vi "UHR-Fleezers Control (host) - Lorentz v2.vi"() -> ()   [LabVIEW 2014] (continued)
          n51 = call "Close.vi"("error in (no error)"=w127, "TTL in"=w124) -> ("error out"=w122:errorcluster)  [unwired: 8 in, 1 out]
        }
        frame Error {
          n52 = call <vilib>:"Simple Error Handler.vi"("error in (no error)"=w205) -> ("error out"=w204:errorcluster)  [unwired: 4 in, 4 out]
        }
      }
      n53 = property on="DAQmx Device Name" class="DAQmxName"("Visible"=FALSE) -> ()  [unwired: 2 in, 2 out]
      n54 = call <vilib>:"Clear Errors.vi"("error in (no error)"=w89) -> ("error out"=w87:errorcluster)  [unwired: 5 in, 1 out]
      n55 = property on="DAQmx Device Name" class="DAQmxName"(error in=w87, "Visible"=TRUE) -> ()  [unwired: 1 in, 2 out]
    }
    frame Disabled {
    }
  }
  n56 = xnode "Open FPGA VI Reference"("resource name"=T24 "RIO0") -> ("FPGA VI Reference Out"=w26:T31, "error out"=w25:errorcluster)  [unwired: 1 in]
  n57 = xnode "Invoke Method"("FPGA VI Reference In"=w26, "error in"=w25) -> ("FPGA VI Reference Out"=w6:T31, "error out"=→"FPGA error out":errorcluster)
  n58 = Subtract(x=w4, y="Maximum Delta\n(MHz)") -> (x-y=w2:dbl)
  n59 = Bundle By Name(cluster=T20 {"Minimum"=60.0, "Maximum"=90.0, "Increment"=1.0} ("Min Max Inc"), "Minimum"=w2, "Maximum"=w4) -> (w1:T20)
  n60 = flat-sequence "Safety limits on RF frequencies and amplitudes (for AOM protection)" {
    tunnel: [w208] -> w17
    tunnel: [w206] -> w19
    tunnel: [w209] -> w20
    tunnel: [w210] -> w18
    tunnel: w1 -> [w208]
    tunnel: T20 {"Minimum"=0.0, "Maximum"=50.0, "Increment"=1.0} ("Data Entry Limits") -> [w206]
    tunnel: w6 -> [w207]
    tunnel: [w207] -> w21
    frame #0 {
      w210 = T20 {"Minimum"=0.0, "Maximum"=40.0, "Increment"=0.1} ("Min Max Inc")
      w209 = T20 {"Minimum"=0.0, "Maximum"=45.0, "Increment"=1.0} ("Data Entry Limits")
      n61 = property on="BD 2 Frequency 1 (MHz)" class="DigNum (strict)"("Data Range"=w210) -> ()  [unwired: 2 in, 2 out]
      n62 = property on="BD 2 Frequency 3 (MHz)" class="DigNum (strict)"("Data Range"=w210) -> ()  [unwired: 2 in, 2 out]
      n63 = property on="BD 2 Frequency 2 (MHz)" class="DigNum (strict)"("Data Range"=w210) -> ()  [unwired: 2 in, 2 out]
      n64 = property on="BD 1 Frequency 1 (MHz)" class="DigNum (strict)"("Data Range"=w208) -> ()  [unwired: 2 in, 2 out]
      n65 = property on="BD 1 Frequency 2 (MHz)" class="DigNum (strict)"("Data Range"=w208) -> ()  [unwired: 2 in, 2 out]
      n66 = property on="BD 1 Frequency 3 (MHz)" class="DigNum (strict)"("Data Range"=w208) -> ()  [unwired: 2 in, 2 out]
      n67 = property on="BD 2 Amplitude 1 (%)" class="DigNum (strict)"("Data Range"=w209) -> ()  [unwired: 2 in, 2 out]
      n68 = property on="BD 2 Amplitude 2 (%)" class="DigNum (strict)"("Data Range"=w209) -> ()  [unwired: 2 in, 2 out]
      n69 = property on="BD 2 Amplitude 3 (%)" class="DigNum (strict)"("Data Range"=w209) -> ()  [unwired: 2 in, 2 out]
      n70 = property on="BD 1 Amplitude 3 (%)" class="DigNum (strict)"("Data Range"=w206) -> ()  [unwired: 2 in, 2 out]
      n71 = property on="BD 1 Amplitude 2 (%)" class="DigNum (strict)"("Data Range"=w206) -> ()  [unwired: 2 in, 2 out]
      n72 = property on="BD 1 Amplitude 1 (%)" class="DigNum (strict)"("Data Range"=w206) -> ()  [unwired: 2 in, 2 out]
      "X RF Frequency Limits (MHz)" <- w208
      "X RF Amplitude Limits (%)" <- w206
      "Y RF Amplitude Limits (%)" <- w209
      "Y RF Frequency Limits (MHz)" <- w210
    }
  }
  n73 = stacked-sequence "Host initialization sequence - order matters!" {
    tunnel: w21 -> [_ w230 w322 _ w379 w388 w455 w479 _ w513]
    tunnel: [_ _ _ _ _ _ _ _ _ w513] -> w10
    tunnel: [_ _ _ _ _ _ _ _ _ w512] -> w23
    tunnel: w20 -> [_ _ _ _ _ _ w453 _ _ _]
    tunnel: w19 -> [_ _ _ _ _ _ w452 _ _ _]
    tunnel: w18 -> [_ _ _ _ _ _ w451 _ _ _]
    tunnel: w17 -> [_ _ _ _ _ _ w432 _ _ _]
    tunnel: [_ _ _ _ _ _ _ _ w507 _] -> _
    frame #0 {
    }
    frame #1 {
      w262 = 10.0 ("y")
      w263 = 32767.0 ("y")
      w247 = 6.0  # clock mult.
      w246 = 49152000.0  # TCXO frequ.
      # "Initialize some FPGA settings"
      n74 = local read "Not-Interlacing Set"() -> (w302:enum32{"Set 1", "Set 2", "Set 3"})
      n75 = local write "Trap Pos FIFO Timeout"(u16 0 ("Trap Pos FIFO Timeout")) -> ()
      n76 = local read "Interlace"() -> (w300:bool)
      n77 = local read "Desired Scan Incr (V)"() -> (w274:dbl)
      n78 = local read "BD 1 Delay (ticks)"() -> (w309:u8)
      n79 = local read "Number Interlace Sets"() -> (w301:u8)
      n80 = local read "BD 2 Delay (Ticks)"() -> (w310:u8)
      n81 = property on="AI Count (ticks)" class="DigNum (strict)"("Val(Sgnl)"="AI Count (ticks)") -> ()  [unwired: 2 in, 2 out]
      n82 = local read "AO1"() -> (w268:dbl)
      n83 = local read "AO2"() -> (w269:dbl)
      n84 = local read "Next trap write delay (ticks)"() -> (w311:u8)
      n85 = local read "Number of scans (MCL)"() -> (w278:u64)
      n86 = local read "Cycles/step (MCL)"() -> (w277:u64)
      n87 = local read "Scan steps (MCL)"() -> (w276:u64)
      n88 = local read "Continuous MCL Scanning"() -> (w279:bool)
      n89 = Multiply(x=w268, y=w263) -> (x*y=w266:dbl)
      n90 = Multiply(x=w269, y=w263) -> (x*y=w264:dbl)
      n91 = Build Array("DIO count 1 (ticks)", "DIO count 2 (ticks)", "DIO count 3 (ticks)") -> (w295:u16[])
      n92 = local read "Fast Scan Dir"() -> (w280:bool)
      n93 = local read "2D or 1D Scan"() -> (w292:bool)
      n94 = local read "N Acq Sets (Traps + Fl.)"() -> (w288:i16)
      n95 = local read "Scan Increment (MHz)"() -> (w251:dbl)
      n96 = Divide(x=w266, y=w262) -> (x/y=w267:dbl)
      n97 = Divide(x=w264, y=w262) -> (x/y=w265:dbl)
      n98 = To Unsigned Byte Integer(number=w302) -> (unsigned 8bit integer=w297:u8)
      n99 = Split 1D Array(array=w295, index=w301) -> (first subarray=w293:u16[])  [unwired: 1 out]
      n100 = Multiply(x=w274, y=32767.0) -> (x*y=w272:dbl)
      n101 = To Word Integer(number=w267) -> (16bit integer=w213:i16)
      n102 = To Word Integer(number=w265) -> (16bit integer=w212:i16)
      n103 = Index Array(array=w295, index=w297) -> (element=w296:u16)
      n104 = Add Array Elements(numeric array=w293) -> (sum=w294:u16)
      n105 = Multiply(x=w246, y=w247) -> (x*y=w248:dbl)
      n106 = Divide(x=w272, y=10.0) -> (x/y=w273:dbl)
      n107 = Select(t=w294, s=w300, f=w296) -> (s? t:f=w303:u16)
      n108 = Not(x=w280) -> (.not. x?=w281:bool)
      n109 = To Word Integer(number=w273) -> (16bit integer=w275:i16)
      n110 = property on="2D or 1D Scan" class="Bool (strict)"("Val(Sgnl)"=w292) -> ()  [unwired: 2 in, 2 out]
      n111 = Divide(x=40000000.0, y="AI Count (ticks)") -> (x/y=w284:dbl)
      n112 = local write "Update Count (MCL)"(w303) -> ()
      n113 = local write "Total Counts (ticks)"(w303) -> ()
      n114 = Divide(x=w284, y="FPGA Ave.") -> (x/y=w283:dbl)
      n115 = local write "AI rate (Hz)"(w284) -> ()
      n116 = Multiply(x=w251, y=1000.0) -> (x*y=w244:dbl)
      n117 = local write "Ave. Rate (Hz)"(w283) -> ()
      n118 = Reciprocal(x=w283) -> (1/x=w282:dbl)
      n119 = Scale By Power Of 2(n=48, x=w244) -> (x*2^n=w243:dbl)
      n120 = local write "Ave. Period (s)"(w282) -> ()
      n121 = Divide(x=w243, y=w248) -> (x/y=w249:dbl)
      n122 = To Quad Integer(1:w249) -> (0:w252:i64)
      n123 = local read "Setpoints (V)"() -> (w237:cluster{"Set 1":dbl, "Set 2":dbl})
      n124 = local read "# Samples/channel"() -> (w259:u32)
      n125 = local read "Feedback On/Off"() -> (w234:cluster{"Set 1":bool, "Set 2":bool})
      n126 = local read "T3 Y (V)"() -> (w217:dbl)
      n127 = local read "T3 X (V)"() -> (w216:dbl)
      n128 = local read "Trap intensity output range"() -> (w227:cluster{"Normal High":i16, "Normal Low":i16})
      n129 = local read "All FB On/Off"() -> (w233:bool)
      n130 = local read "Number of F/B Scans (AOD)"() -> (w258:u16)
      n131 = local read "Trap Intensity PID Gains"() -> (w226:T11)
      n132 = local read "Cycles/step (AOD)"() -> (w254:u64)
      n133 = local read "Scan steps (AOD)"() -> (w253:u64)
      n134 = Multiply(x=w253, y=w254) -> (x*y=w255:u64)
      n135 = Multiply(x=w255, y=u64 2) -> (x*y=w257:u64)
      n136 = Multiply(x=w257, y=w258) -> (x*y=w260:u64)
      n137 = Multiply(x=3276.7, y=w237) -> (x*y=w238:cluster{"Set 1":dbl, "Set 2":dbl})
      n138 = local read "Scan BD"() -> (w242:bool)
      n139 = Multiply(x=w217, y=32767.0) -> (x*y=w223:dbl)
      n140 = And(x=w234, y=w233) -> (x .and. y?=w235:cluster{"Set 1":bool, "Set 2":bool})
      n141 = To Word Integer(number=w238) -> (16bit integer=w239:cluster{"Set 1":i16, "Set 2":i16})
      n142 = Multiply(x=w216, y=32767.0) -> (x*y=w220:dbl)
      n143 = local read "Sets to FIFO (Traps)"() -> (w305:T19)
      n144 = Divide(x=w260, y=w259) -> (x/y=w261:dbl)
      n145 = Unbundle By Name(w235) -> ("Set 1"=w231:bool, "Set 2"=w232:bool)
      n146 = Unbundle By Name(w239) -> ("Set 1"=w240:i16, "Set 2"=w241:i16)
      n147 = Divide(x=w223, y=10.0) -> (x/y=w224:dbl)
      n148 = Divide(x=w220, y=10.0) -> (x/y=w219:dbl)
      n149 = To Word Integer(number=w224) -> (16bit integer=w215:i16)
      n150 = To Word Integer(number=w219) -> (16bit integer=w214:i16)
      n151 = local read "FPGA error out"() -> (w229:errorcluster)
      n152 = local write "Data points/scan (f/b)"(w257) -> ()
      n153 = local write "Data points/scans"(w260) -> ()
      n154 = local write "N sets should be saved"(w261) -> ()
      n155 = Unbundle By Name(w305) -> ("Set 1"=w306:bool, "Set 2"=w307:bool, "Set 3"=w308:bool)
      n156 = xnode "Read/Write Control"("FPGA VI Reference In"=w230, "error in"=w229, "ai count"="AI Count (ticks)", "Interlace ON/OFF"=w300, "Number Interlace Cycles"=w301, "Set 1"=w306, "Set 2"=w307, "Set 3"=w308, "FB On/Off Set 1"=w231, "FB On/Off Set 2"=w232, "Interlace Off Parameters"=w302, "FB Setpoint Set 1"=w240, "FB Setpoint Set 2"=w241, "AO4"=w215, "AO5"=w214, "FB Gains"=w226, "FB output range"=w227, "Cycles per step"=w254, "Scan BD"=w242, "Number of scans"=w258, "Scan steps"=w253, "Scan freq.  increment"=w252, "AO1"=w213, "AO2"=w212, "Scan freq.  increment (MCL)"=w275, "Scan steps (MCL)"=w276, "Cycles per step (MCL)"=w277, "Number of scans (MCL)"=w278, "MCL count"=w303, "Cont. Scan (MCL)"=w279, "MCL Scan Axis"=w281, "1D or 2D Scan?"=w292, "N of AI1 Int Acq Sets"=w288, "Amp switch delay"="Amp switch delay", "Swap F1 and F2"="Swap F1 and F2", "APD to FIFO"=FALSE, "DIO count 1 (ticks)"="DIO count 1 (ticks)", "DIO count 2 (ticks)"="DIO count 2 (ticks)", "DIO count 3 (ticks)"="DIO count 3 (ticks)", "BD 1 Delay (ticks)"=w309, "BD 2 Delay (Ticks)"=w310, "Next trap write delay (ticks)"=w311) -> ("error out"=w228:errorcluster)  [unwired: 1 out]
      n157 = local write "FPGA error out"(w228) -> ()
    }
    frame #2 {
      # "Initialize some more FPGA settings"
      n158 = local read "Trap Pos FB Monitor\nT1 or T2"() -> (w333:bool)
      n159 = local read "Trap Pos FB Negate Action"() -> (w334:bool)
      n160 = local read "Trap Pos. FB Offset Factor"() -> (w335:i64)
      n161 = local read "Trap Pos. FB Mult Factor"() -> (w336:i64)
      n162 = local read "Trap Pos. AI1 X Pre-scale"() -> (w338:u16)
      n163 = local read "Trap Pos FB Int Count"() -> (w340:u16)
      n164 = local read "Green Laser ON"() -> (w312:bool)
      n165 = local read "Neg. TTrig FPGA"() -> (w341:bool)
      n166 = local read "Trap Pos. FB Range"() -> (w317:T15)
      n167 = local read "Trap Pos. FB Gains"() -> (w318:T14)
      n168 = local read "Dynamic Force FB (ronen)"() -> (w319:bool)
      n169 = Multiply(x="Green Intensity % (FB OFF)", y=655.35) -> (x*y=w327:dbl)
      n170 = Multiply(x="Red FB Setpoint (mV)", y=3.2767) -> (x*y=w349:dbl)
      n171 = Multiply(x="Red Intensity % (FB OFF)", y=655.35) -> (x*y=w353:dbl)
      n172 = Unbundle By Name("Red FB Gains") -> ("proportional gain (Kc)"=w358:i16, "integral gain (Kc*Ts/Ti)"=w359:i16, "derivative gain (Kc*Td/Ts)"=w360:i16)
      n173 = Multiply(x="Green FB Setpoint (mV)", y=3.2767) -> (x*y=w330:dbl)
      n174 = To Unsigned Word Integer(number=w327) -> (unsigned 16bit integer=w329:u16)
      n175 = To Unsigned Word Integer(number=w353) -> (unsigned 16bit integer=w356:u16)
      n176 = To Word Integer(number=w349) -> (16bit integer=w352:i16)
      n177 = local read "Differential FB?"() -> (w343:bool)
      n178 = To Word Integer(number=w330) -> (16bit integer=w332:i16)
      n179 = local read "Laser interlacing mode"() -> (w315:enum32{"Laser ON", "Laser OFF", "Interlace"})
      n180 = local read "Invert laser interlacing"() -> (w316:bool)
      n181 = Unbundle By Name("Green FB Gains") -> ("proportional gain (Kc)"=w346:i16, "integral gain (Kc*Ts/Ti)"=w347:i16, "derivative gain (Kc*Td/Ts)"=w348:i16)
      n182 = Select(t=w315, s=w312, f=enum32{"Laser ON", "Laser OFF", "Interlace"}."Laser OFF" ("Green laser mode")) -> (s? t:f=w314:enum32{"Laser ON", "Laser OFF", "Interlace"})
      n183 = local read "FPGA error out"() -> (w320:errorcluster)
      n184 = xnode "Read/Write Control"("FPGA VI Reference In"=w322, "error in"=w320, "Invert GI"=w316, "Invert GI 2"=w316, "Invert RI"=w316, "Invert RI 2"=w316, "Operating Mode"=w314, "Operating Mode 2"=w314, "Red Laser Operating Mode"=w314, "RI Operating Mode 2"=w314, "P3"=w346, "I3"=w347, "D3"=w348, "Green FB Setpoint"=w332, "Green FB On/Off"="Green FB On/Off", "Current Out"=w329, "Green int current ON count adj"="Green int current ON count adj", "Trap Pos FB Monitor T1 or T2"=w333, "Trap Pos FB Negate Action"=w334, "Trap Pos. FB Offset Factor"=w335, "Trap Pos. FB Mult Factor"=w336, "Force feedback"=FALSE, "AI1 X Scale"=w338, "Trap Pos to FIFO"=TRUE, "Trap Pos FB Int Count"=w340, "TTrig Negate Pos"=w341, "FB Trig Integrate"="FB Trig Integrate", "Diff FB Measurement?"=w343, "Negate Diff?"="Negate Diff?", "Trap pos. FB Range"=w317, "Trap Pos. FB Gains"=w318, "Red FB Setpoint"=w352, "RI Current Out"=w356, "P4"=w358, "I4"=w359, "D4"=w360, "Red FB On/Off"="Red FB On/Off", "Dynamic Force FB (Ronen)"=w319) -> ("error out"=w321:errorcluster)  [unwired: 1 out]
      n185 = local write "FPGA error out"(w321) -> ()
    }
    frame #3 {
      # "Initialize more settings. Should stop using event loops to initialize."
      # "What are these?"
      n186 = local write "Offset (nm)"(0.0 ("Offset (nm)")) -> ()
      n187 = local write "Bead Mean (nm)"(0.0 ("Bead Mean (nm)")) -> ()
      n188 = stacked-sequence {
        frame #0 {
          w364 = T33."empty" ("mode")
          # "Clear external fluorescence triggering FIFO"
          # "APD loop counts"
          # "Fluorescence loop counts (rates)"
          n189 = local read "APD Integration Time (s)"() -> (w366:dbl)
          n190 = local read "Interlace ON count"() -> (w367:u16)
          n191 = call "Smart Buffer (DBL) 1.vi"("mode"=w364) -> ()  [unwired: 5 in, 6 out]
          n192 = call "Smart Buffer (DBL) 2.vi"("mode"=w364) -> ()  [unwired: 5 in, 6 out]
          n193 = property on="APD Integration Time (s)" class="DigNum (strict)"("Val(Sgnl)"=w366) -> ()  [unwired: 2 in, 2 out]
          n194 = property on="Interlace ON count" class="DigNum (strict)"("Val(Sgnl)"=w367) -> ()  [unwired: 2 in, 2 out]
          "Number of APDs" <- 3.0 ("Number of APDs")
        }
        frame #1 {
          # "Number of APDs affects\nAPD DMA transfer"
          # "General settings for all lasers:"
          # "And includes all laser\nON/OFF settings"
          # "Fluorescent lasers settings:"
          # "Blue laser settings:"
          n195 = local read "Laser interlacing mode"() -> (w369:enum32{"Laser ON", "Laser OFF", "Interlace"})
          n196 = local read "Invert laser interlacing"() -> (w368:bool)
          n197 = local read "Blue FB On/Off"() -> (w370:bool)
          n198 = property on="Blue FB On/Off" class="Bool (strict)"("Val(Sgnl)"=w370) -> ()  [unwired: 2 in, 2 out]
          n199 = property on="Invert laser interlacing" class="Bool (strict)"("Val(Sgnl)"=w368) -> ()  [unwired: 2 in, 2 out]
          n200 = property on="Laser interlacing mode" class="RadioBtnsControl (strict)"("Val(Sgnl)"=w369) -> ()  [unwired: 2 in, 2 out]
        }
        frame #2 {
          w371 = path "C:/Home/Bustamante Lab/Comstock-LabView-Link.udl" ("connection information")
          # "Database link changed by Ronen - not clear if it matter for the program."
          # "Initialize the database connection"
          n201 = disable-structure shown="Disabled" {
            disable-tunnel: [w374 _] -> w372
            disable-tunnel: w371 -> [w373 _]
            frame Disabled {
              n202 = call-poly <vilib>:"DB Tools Open Connection.vi"("connection information"=w373) -> ("connection reference"=w374:T21)  [unwired: 7 in, 1 out]
            }
            frame Enabled {
            }
          }
          "connection reference" <- w372
          n203 = local write "connection reference"(w372) -> ()
          n204 = local write "Database link"(w371) -> ()
        }
        frame #3 {
          # "Load active calibration to fpga"
          n205 = local read "Base N trap periods"() -> (w376:u32)
          n206 = local read "T1 Osc Enable"() -> (w375:bool)
          n207 = property on="T1 Osc Enable" class="Bool (strict)"("Val(Sgnl)"=w375) -> ()  [unwired: 2 in, 2 out]
          n208 = property on="Base N trap periods" class="DigNum (strict)"("Val(Sgnl)"=w376) -> ()  [unwired: 2 in, 2 out]
        }
      }
    }
    frame #4 {
      # "Set FIFO size and run FPGA"
      n209 = local read "FPGA error out"() -> (w378:errorcluster)
      n210 = xnode "Invoke Method"("FPGA VI Reference In"=w379, "error in"=w378, "Requested Depth"="Trap AI FIFO Depth") -> ("FPGA VI Reference Out"=w383:T31, "error out"=w384:errorcluster)  [unwired: 1 out]
      n211 = xnode "Invoke Method"("FPGA VI Reference In"=w383, "error in"=w384, "Requested Depth"="Trap Position FIFO Depth") -> ("FPGA VI Reference Out"=w381:T31, "error out"=w380:errorcluster)  [unwired: 1 out]
      n212 = xnode "Invoke Method"("FPGA VI Reference In"=w381, "error in"=w380) -> ("error out"=w377:errorcluster)  [unwired: 1 in, 1 out]
      n213 = local write "FPGA error out"(w377) -> ()
    }
    frame #5 {
      # "Adjust FPGA timing loop phases"
      n214 = flat-sequence "Initial FPGA Loop Relative Phase Adjustment" {
        tunnel: "Initial Phase Adjustment (AI1)" -> [w418]
        tunnel: "Initial Phase Adjustment (GI)" -> [w417]
        tunnel: "Initial Phase Adj. (MCL)" -> [w416]
        tunnel: [w419] -> w403
        tunnel: [w415] -> w402
        tunnel: "Initial Phase Adjustment (APD Acq)" -> [w414]
        tunnel: "Initial Phase Adjustment (APD 1 Gate)" -> [w413]
        tunnel: "Initial Phase Adjustment (Green FB)" -> [w412]
        tunnel: "Initial Phase Adjustment (GI) 2" -> [w411]
        tunnel: "Initial Phase Adjustment (APD 2 Gate)" -> [w410]
        tunnel: "Initial Phase Adjustment (RI)" -> [w409]
        tunnel: "Initial Phase Adjustment (BI DO)" -> [w408]
        tunnel: "Initial Phase Adjustment (BI AO)" -> [w407]
        tunnel: "Initial Phase Adjustment (APD 3 Gate)" -> [w406]
        tunnel: w388 -> [w405]
        tunnel: w403 -> [w421]
        tunnel: [w422] -> w401
        tunnel: w402 -> [w422]
        tunnel: [w421] -> w400
        tunnel: w401 -> [w426]
        tunnel: w400 -> [w425]
        tunnel: [w423] -> w387
        frame #0 {
          n215 = local read "FPGA error out"() -> (w404:errorcluster)
          n216 = xnode "Read/Write Control"("FPGA VI Reference In"=w405, "error in"=w404, "Phase count adjustment"=w418, "Phase count adjustment (GI)"=w417, "Phase count adjustment (MCL)"=w416, "Phase Count Adjustment (APD Acq)"=w414, "Phase count adjustment (APD 1 Gate)"=w413, "Phase count adjustment (APD 2 Gate)"=w410, "Phase count adjustment (Green FB)"=w412, "Phase count adjustment (GI) 2"=w411, "Phase count adjustment (RI)"=w409, "Phase count adjustment (BI AO)"=w407, "Phase count adjustment (BI D)"=w408, "Phase count adjustment (APD 3 Gate)"=w406) -> ("FPGA VI Reference Out"=w415:T31, "error out"=w419:errorcluster)
        }
        frame #1 {
          n217 = Wait (ms)(milliseconds to wait=u32 100) -> ()  [unwired: 1 out]
        }
        frame #2 {
          w424 = TRUE
          n218 = xnode "Read/Write Control"("FPGA VI Reference In"=w426, "error in"=w425, "+ phase"=w424, "+ phase (GI)"=w424, "+ phase (MCL)"=w424, "+ phase (APD Acq)"=w424, "+ phase (APD 1 Gate)"=w424, "+ phase (APD 2 Gate)"=w424, "+ phase (Green FB)"=w424, "+ phase (GI) 2"=w424, "+ phase (RI)"=w424, "+ phase (BI AO)"=w424, "+ phase (BI D)"=w424, "+ phase (APD 3 Gate)"=w424) -> ("error out"=w423:errorcluster)  [unwired: 1 out]
        }
      }
      n219 = local write "FPGA error out"(w387) -> ()
    }
    frame #6 {
      w440 = 6.0  # clock mult.
      w439 = 49152000.0  # TCXO frequ.
      w444 = 6.0  # clock mult.
      w445 = 49152000.0  # TCXO frequ.
      # "Added by ronen - definition of \nlimit frequencies when using dynamic feedback"
      # "Initialize trap RF synth board and set initial frequencies and amplitudes"
      n220 = local read "FPGA error out"() -> (w454:errorcluster)
      n221 = call "Initialize RF boards - interlace 3.vi"("error in"=w454, "FPGA VI Reference In"=w455) -> ("error out"=w456:errorcluster, "FPGA VI Reference Out"=w476:T31)
      n222 = call "set RF board frequency - interlace.vi"("Board 2 Frequency Limits"=w451, "Board 1 Frequency Limits"=w432, "error in"=w456, "FPGA VI Reference In"=w476, "Board 2 Frequency 3 (MHz)"="BD 2 Frequency 3 (MHz)", "Board 1 Frequency 3 (MHz)"="BD 1 Frequency 3 (MHz)", "Board 2 Frequency 2 (MHz)"="BD 2 Frequency 2 (MHz)", "Board 2 Frequency 1 (MHz)"="BD 2 Frequency 1 (MHz)", "Board 1 Frequency 2 (MHz)"="BD 1 Frequency 2 (MHz)", "Board 1 Frequency 1  (MHz)"="BD 1 Frequency 1 (MHz)") -> ("error out"=w459:errorcluster, "FPGA VI Reference Out"=w431:T31)
      n223 = Unbundle By Name(w432) -> ("Maximum"=w442:dbl, "Minimum"=w433:dbl)
      n224 = call "set RF board amplitude - interlace.vi"("Board 2 Amplitude Limits"=w453, "Board 1 Amplitude Limits"=w452, "error in"=w459, "FPGA VI Reference In"=w431, "Board 2 Amplitude 3 (%)"="BD 2 Amplitude 3 (%)", "Board 1 Amplitude 3 (%)"="BD 1 Amplitude 3 (%)", "Board 2 Amplitude 2 (%)"="BD 2 Amplitude 2 (%)", "Board 2 Amplitude 1 (%)"="BD 2 Amplitude 1 (%)", "Board 1 Amplitude 2 (%)"="BD 1 Amplitude 2 (%)", "Board 1 Amplitude 1 (%)"="BD 1 Amplitude 1 (%)") -> ("error out"=w428:errorcluster)  [unwired: 1 out]
      n225 = Multiply(x=w433, y=1000000.0) -> (x*y=w437:dbl)
      n226 = Multiply(x=w442, y=1000000.0) -> (x*y=w447:dbl)
      n227 = Scale By Power Of 2(n=48, x=w437) -> (x*2^n=w435:dbl)
      n228 = Subtract(x="BD 1 Frequency 1 (MHz)", y="BD 1 Frequency 2 (MHz)") -> (x-y=w466:dbl)
      n229 = Subtract(x="BD 2 Frequency 1 (MHz)", y="BD 2 Frequency 2 (MHz)") -> (x-y=w467:dbl)
      n230 = Scale By Power Of 2(n=48, x=w447) -> (x*2^n=w449:dbl)
      n231 = Multiply(x=w439, y=w440) -> (x*y=w441:dbl)
      n232 = Multiply(x=w445, y=w444) -> (x*y=w443:dbl)
      n233 = Square(x=w467) -> (x^2=w469:dbl)
      n234 = Square(x=w466) -> (x^2=w468:dbl)
      n235 = Divide(x=w435, y=w441) -> (x/y=w436:dbl)
      n236 = Divide(x=w449, y=w443) -> (x/y=w448:dbl)
      n237 = Add(x=w468, y=w469) -> (x+y=w470:dbl)
      n238 = To Unsigned Quad Integer(1:w436) -> (0:w429:u64)
      n239 = To Unsigned Quad Integer(1:w448) -> (0:w430:u64)
      n240 = Square Root(x=w470) -> (sqrt(x)=w471:dbl)
      n241 = local write "Trap Delta (MHz)"(w471) -> ()
      n242 = xnode "Read/Write Control"("FPGA VI Reference In"=w431, "error in"=w428, "FB Max Frequency"=w430, "FB Min frequency"=w429) -> ("error out"=w427:errorcluster)  [unwired: 1 out]
      n243 = local write "FPGA error out"(w427) -> ()
    }
    frame #7 {
      n244 = local read "FPGA error out"() -> (w478:errorcluster)
      n245 = flat-sequence {
        tunnel: [w493] -> w483
        tunnel: [w492] -> w482
        tunnel: w479 -> [w485]
        tunnel: w478 -> [w484]
        tunnel: [w497] -> w481
        tunnel: w483 -> [w497]
        tunnel: [w496] -> w480
        tunnel: w482 -> [w496]
        tunnel: w481 -> [w505]
        tunnel: w480 -> [w504]
        tunnel: [w499] -> w477
        frame #0 {
          w486 = FALSE ("Retract Pump 3")
          n246 = xnode "Read/Write Control"("FPGA VI Reference In"=w485, "error in"=w484, "Direct RF Box  Communication"=FALSE) -> ("FPGA VI Reference Out"=w493:T31, "error out"=w492:errorcluster)
          n247 = local read "Trap 1 (ON/OFF)"() -> (w487:bool)
          n248 = local write "Saving..."(FALSE ("Saving Data")) -> ()
          n249 = local write "Stop All"(FALSE ("Stop All")) -> ()
          n250 = local write "Retract Pump 1"(w486) -> ()
          n251 = local write "Retract Pump 3"(w486) -> ()
          n252 = local write "Index"(1.0 ("Index")) -> ()
          n253 = property on="Trap 1 ON" class="Bool (strict)"("Value"=w487) -> ()  [unwired: 2 in, 2 out]
          "Manipulating Trap" <- FALSE ("Manipulating Trap")
        }
        frame #1 {
          n254 = local read "Trap 2 (ON/OFF)"() -> (w495:bool)
          n255 = Wait (ms)(milliseconds to wait=u32 10) -> ()  [unwired: 1 out]
          n256 = property on="Trap 2 ON" class="Bool (strict)"("Val(Sgnl)"=w495) -> ()  [unwired: 2 in, 2 out]
        }
        frame #2 {
          n257 = xnode "Read/Write Control"("FPGA VI Reference In"=w505, "error in"=w504, "FPGA Controls  RF Box"=TRUE ("Direct RF Box  Communication")) -> ("error out"=w499:errorcluster)  [unwired: 1 out]
          n258 = local read "Scan Range (nm)"() -> (w500:dbl)
          n259 = call "Update messages.vi"("Message to add"="UHR-Fleezers ready.", "Old message string"="") -> ("New message string"=w503:string)
          n260 = local write "Messages"(w503) -> ()
          n261 = property on="Scan Range (nm)" class="DigNum (strict)"("Val(Sgnl)"=w500) -> ()  [unwired: 2 in, 2 out]
        }
      }
      n262 = local write "FPGA error out"(w477) -> ()
    }
    frame #8 {
      n263 = call "hamilton_controller.vi"("action"=T32."CONNECT") -> ("error out"=w510:errorcluster)  [unwired: 9 in, 1 out]
      n264 = call "hamilton_controller.vi"("error in"=w510, "action"=T32."INITIALIZE VALVES") -> ("error out"=w507:errorcluster)  [unwired: 8 in, 1 out]
    }
    frame #9 {
      # "Wait 5 s for all the event loops still being executed to finish."
      n265 = Wait (ms)(milliseconds to wait=u32 5000) -> ()  [unwired: 1 out]
      n266 = local read "FPGA error out"() -> (w512:errorcluster)
    }
  }
  n267 = disable-structure shown="Disabled" {
    disable-tunnel: [w545 _] -> w55
    disable-tunnel: [w542 _] -> w44
    disable-tunnel: [w541 _] -> w43
    disable-tunnel: [w536 _] -> w39
    disable-tunnel: [w535 _] -> w38
    disable-tunnel: [w534 _] -> w37
    disable-tunnel: [w533 _] -> w36
    disable-tunnel: [w530 _] -> w28
    disable-tunnel: [w525 _] -> w9
    disable-tunnel: [w518 _] -> w8
    disable-tunnel: [w515 _] -> w7
    frame Disabled {
      w517 = u16 20 items=["1.0"=10, "1.5"=15, "2.0"=20] ("stop bits (10: 1 bit)")
      w528 = u16 20 items=["1.0"=10, "1.5"=15, "2.0"=20] ("stop bits (10: 1 bit)")
      w531 = u16 10 items=["1.0"=10, "1.5"=15, "2.0"=20] ("stop bits (10: 1 bit)")
      w537 = u16 20 items=["1.0"=10, "1.5"=15, "2.0"=20] ("stop bits (10: 1 bit)")
      w539 = u16 20 items=["1.0"=10, "1.5"=15, "2.0"=20] ("stop bits (10: 1 bit)")
      w543 = u16 20 items=["1.0"=10, "1.5"=15, "2.0"=20] ("stop bits (10: 1 bit)")
      # "Bottom 1 Harvard"
      # "Top 3 Harvard"
      # "Center Harvard"
      n268 = call-poly "VISA Configure Serial Port"("VISA resource name"=refnum<visa-resource-name> "COM2", "baud rate (9600)"=u32 9600, "stop bits (10: 1 bit)"=w528) -> ("VISA resource name out"=w518:refnum<visa-resource-name>, "error out"=→"Preamp Error Out":errorcluster)  [unwired: 4 in, 7 out]
      n269 = call-poly "VISA Configure Serial Port"("VISA resource name"=refnum<visa-resource-name> "COM2", "baud rate (9600)"=u32 9600, "stop bits (10: 1 bit)"=w517) -> ("VISA resource name out"=w515:refnum<visa-resource-name>)  [unwired: 4 in, 8 out]
      n270 = call-poly "VISA Configure Serial Port"("VISA resource name"=refnum<visa-resource-name> "COM7", "baud rate (9600)"=u32 115200, "stop bits (10: 1 bit)"=w531) -> ("VISA resource name out"=w530:refnum<visa-resource-name>, "error out"=w529:errorcluster)  [unwired: 4 in, 7 out]
      n271 = call-poly "VISA Configure Serial Port"("VISA resource name"=refnum<visa-resource-name> "COM5", "baud rate (9600)"=u32 115200, "stop bits (10: 1 bit)"=w537) -> ("VISA resource name out"=w534:refnum<visa-resource-name>, "error out"=w533:errorcluster)  [unwired: 4 in, 7 out]
      n272 = call-poly "VISA Configure Serial Port"("VISA resource name"=refnum<visa-resource-name> "COM4", "baud rate (9600)"=u32 115200, "stop bits (10: 1 bit)"=w539) -> ("VISA resource name out"=w536:refnum<visa-resource-name>, "error out"=w535:errorcluster)  [unwired: 4 in, 7 out]
      n273 = call-poly "VISA Configure Serial Port"("VISA resource name"=refnum<visa-resource-name> "COM6", "baud rate (9600)"=u32 115200, "stop bits (10: 1 bit)"=w543) -> ("VISA resource name out"=w541:refnum<visa-resource-name>, "error out"=w542:errorcluster)  [unwired: 4 in, 7 out]
      n274 = call-poly "VISA Configure Serial Port"("VISA resource name"=refnum<visa-resource-name> "COM1") -> ("VISA resource name out"=w525:refnum<visa-resource-name>, "error out"=w545:errorcluster)  [unwired: 5 in, 8 out]
      "Stage Control Serial Error" <- w545
      n275 = local write "Blue Error Out"(w529) -> ()
    }
    frame Enabled {
    }
  }
  n276 = call "IMAQ Create"("Image Name"="APD 1 Image", "Image Type"=w32) -> ("New Image"=w49:T2)  [unwired: 3 in, 1 out]
  n277 = call "IMAQ Create"("Image Name"="APD 2 Image", "Image Type"=w32) -> ("New Image"=w48:T2)  [unwired: 3 in, 1 out]
  n278 = call "IMAQ Create"("Image Name"="APD 3 Image", "Image Type"=w32) -> ("New Image"=w31:T2)  [unwired: 3 in, 1 out]
  n279 = call "IMAQ Create"("Image Name"="Det. X Image", "Image Type"=w32) -> ("New Image"=w47:T2)  [unwired: 3 in, 1 out]
  n280 = call "IMAQ Create"("Image Name"="Det. Y Image", "Image Type"=w32) -> ("New Image"=w46:T2)  [unwired: 3 in, 1 out]
  n281 = Bundle("New Image"=w49, "New Image"=w48, "New Image"=w31, "New Image"=w47, "New Image"=w46) -> (w45:T34)  [unwired: 1 in]
  n282 = node-c288() -> (w52:T35)  [unwired: 4 in]
  n283 = timed-loop "Run Scripts, including: stage motion" {
    tunnel: w55 -> [w556]
    tunnel: w9 -> [w557]
    tunnel: [w557] -> w54
    tunnel: [w556] -> w53
    timing: w52 -> [_]
    timing-out: [_] -> w51
    tunnel: w43 -> [w555]
    tunnel: w44 -> [w554]
    tunnel: w39 -> [w551]
    tunnel: w38 -> [w550]
    tunnel: w37 -> [w552]
    tunnel: w36 -> [w553]
    tunnel: w28 -> [w549]
    tunnel: w21 -> [w548]
    tunnel: w8 -> [w547]
    tunnel: w7 -> [w546]
    stop <- w558 stop-if-true
    n284 = node-c288() -> ()  [unwired: 1 in, 1 out]
    n285 = event shown="[17] \"Got Bead 1\": Value Change" {
      selector: _ -> [_ _ _ _ _ _ _ _ _ _ _ _ _ _ _ _ _ _ _ _ _ _ _ _ _ _ _ _]
      dyn-events: _ -> [_ _ _ _ _ _ _ _ _ _ _ _ _ _ _ _ _ _ _ _ _ _ _ _ _ _ _ _]
      timeout: _ -> [_ _ _ _ _ _ _ _ _ _ _ _ _ _ _ _ _ _ _ _ _ _ _ _ _ _ _ _]
      tunnel: ["Set Position" "Move to Position" _ _ _ _ _ _ "Read Harvard" _ _ _ _ _ _ _ _ "Got Bead 1" "Force FB Data\nScript" _ "Got Bead 2" _ "Take Stepping Data" _ "Take Detection Laser\nImage" _ _ _] -> _
      tunnel: [_ _ _ _ _ _ _ _ _ _ _ _ _ _ _ _ _ _ _ _ _ _ _ _ _ _ w1485 _] -> w558
      tunnel: w556 -> [w577 w585 w598 w628 _ _ _ _ _ w765 w799 w825 w857 w946 w975 w1107 w1134 _ w1176 _ _ _ _ _ _ _ _ _]
      tunnel: w557 -> [w578 w586 w599 w629 _ _ _ _ _ w766 w800 w826 w858 w947 w976 w1108 w1135 _ w1177 _ _ _ _ _ _ _ _ _]
      tunnel: w555 -> [_ _ _ _ _ _ _ _ w750 _ _ _ _ _ _ _ _ _ _ _ _ _ _ _ _ _ _ _]
      tunnel: w554 -> [_ _ _ _ _ _ _ _ w749 _ _ _ _ _ _ _ _ _ _ _ _ _ _ _ _ _ _ _]
      tunnel: w553 -> [_ _ _ _ _ _ _ _ _ _ _ _ _ _ _ _ _ _ _ _ _ _ _ _ _ _ _ _]
      tunnel: w552 -> [_ _ _ _ _ _ _ _ _ _ _ _ _ _ _ _ _ _ _ _ _ _ _ _ _ _ _ _]
      tunnel: w551 -> [_ _ _ _ _ _ _ _ _ _ _ _ _ _ _ _ _ _ _ _ _ _ _ _ _ _ _ _]
      tunnel: w550 -> [_ _ _ _ _ _ _ _ _ _ _ _ _ _ _ _ _ _ _ _ _ _ _ _ _ _ _ _]
      tunnel: w549 -> [_ _ _ _ w656 w663 w691 w710 _ _ _ _ _ _ _ _ _ _ _ _ _ _ _ _ _ _ w1484 _]
      tunnel: w548 -> [_ _ _ _ _ _ _ _ _ _ _ _ _ _ _ _ _ _ _ _ _ _ _ _ _ w1351 _ _]
      tunnel: w547 -> [_ _ _ _ _ _ _ _ _ _ _ _ _ _ _ _ _ _ _ _ _ _ _ _ _ _ _ w1495]
      tunnel: w546 -> [_ _ _ _ _ _ _ _ _ _ _ _ _ _ _ _ _ _ _ _ _ _ _ _ _ _ _ w1490]
      tunnel: [_ _ _ _ _ _ _ _ _ _ _ _ _ _ _ _ _ _ _ _ _ "Get New Beads" _ _ _ _ _ _] -> _
      event "Set Position", "Set Position 2", "Set Position 3", "Set Position 4", "Set Position 5", "Set Position 1", "Set Position 6": Value Change {
        n286 = event-data() -> ()  [unwired: 1 in, 5 out]
        n287 = Build Array("Set Position 1", "Set Position 2", "Set Position 3", "Set Position 4", "Set Position 5", "Set Position 6") -> (w576:bool[])
        n288 = Boolean Array To Number(Boolean array=w576) -> (number=w575:u32)
        n289 = Logarithm Base 2(1:w575) -> (0:w567:dbl)
        n290 = call "Read Stage Position.vi"("error in"=w577, "VISA resource name in"=w578) -> ("Current Position"=w582:cluster{dbl, dbl, dbl}, "error out"=w581:errorcluster)  [unwired: 2 out]
        n291 = Decrement(x="Position") -> (x-1=w565:dbl)
        n292 = Greater Or Equal?(x=w567, y=0.0) -> (x >= y?=w568:bool)
        n293 = Cluster To Array(cluster=w582) -> (array=w579:dbl[])
        n294 = local write "Stage Control Serial Error"(w581) -> ()
        n295 = Select(t=w567, s=w568, f=w565) -> (s? t:f=w564:dbl)
        n296 = Increment(x=w564) -> (x+1=w563:dbl)
        n297 = Build Array (concatenate)(w563, w579) -> (w562:dbl[])
        n298 = Replace Array Subset(array="Saved Stage Positions", new element=w562, index (row)=w564) -> (w580:dbl[][])  [unwired: 1 in]
        n299 = local write "Saved Stage Positions"(w580) -> ()
      }
      event "Move to Position": Value Change {
        n300 = event-data() -> ()  [unwired: 1 in, 5 out]
        n301 = flat-sequence {
          tunnel: w586 -> [w590]
          tunnel: w585 -> [w589]
          frame #0 {
            n302 = local read "Saved Stage Positions"() -> (w592:dbl[][])
            n303 = local read "Position"() -> (w591:dbl)
            n304 = local write "Stage Moving"(TRUE ("Stage Moving")) -> ()
            n305 = call "move to saved stage position.vi"("error in"=w589, "Stage VISA resource name in"=w590, "Position"=w591, "Saved Stage Positions"=w592) -> ("error out"=w588:errorcluster)  [unwired: 1 out]
            n306 = local write "Stage Control Serial Error"(w588) -> ()
          }
          frame #1 {
            n307 = call <vilib>:"Beep.vi"() -> ()  [unwired: 3 in, 9 out]
            n308 = local write "Stage Moving"(FALSE ("Stage Moving")) -> ()
          }
        }
      }
      event "Move Cap. 1 (DNA Bottom)": Value Change {
        n309 = event-data() -> ()  [unwired: 1 in, 5 out]
        n310 = local write "Move Cap. 1 (DNA Bottom)"(FALSE ("Move Cap. 1 (DNA Right)")) -> ()
        n311 = flat-sequence {
          tunnel: w598 -> [w601]
          tunnel: w599 -> [w602]
          tunnel: [w602] -> w596
          tunnel: [w601] -> w595
          tunnel: w596 -> [w604]
          tunnel: w595 -> [w603]
          frame #0 {
            n312 = property on="Sample Channel\nFlow" class="Bool (strict)"("Val(Sgnl)"="Cap 1 Samp Flow ON") -> ()  [unwired: 2 in, 2 out]
          }
          frame #1 {
            n313 = local read "Saved Stage Positions"() -> (w614:dbl[][])
            n314 = local write "Stage Moving"(TRUE ("Stage Moving")) -> ()
            n315 = Array Subset(array=w614, index (row)=0 ("index"), length (row)=1 ("length"), index (col)=1 ("index"), length (col)=3 ("length")) -> (w611:dbl[][])
            n316 = Reshape Array(w611, 3 ("dimension size")) -> (w609:dbl[])
            n317 = Array To Cluster(array=w609) -> (cluster=w608:cluster{"[0]":dbl, "[1]":dbl, "[2]":dbl})
            n318 = call "Set Stage Position.vi"("Position"=w608, "error in"=w603, "VISA resource name in"=w604) -> ("error out"=w607:errorcluster)  [unwired: 2 out]
            n319 = local write "Stage Control Serial Error"(w607) -> ()
          }
          frame #2 {
            n320 = local write "Stage Moving"(FALSE ("Stage Moving")) -> ()
            n321 = case shown="True" "Cap 1 Flow ON" {
              frame False {
              }
              frame True {
                n322 = property on="Inject Pump 1" class="Bool (strict)"("Val(Sgnl)"=TRUE ("Value (Signaling)")) -> ()  [unwired: 2 in, 2 out]
              }
            }
            n323 = call <vilib>:"Beep.vi"() -> ()  [unwired: 3 in, 9 out]
          }
          frame #3 {
            n324 = property on="Sample Channel\nFlow" class="Bool (strict)"("Val(Sgnl)"=FALSE ("Value (Signaling)")) -> ()  [unwired: 2 in, 2 out]
            n325 = local read "Cap. 2 BD T1?\n(ADig T1, DNA T2)"() -> (w621:bool)
            n326 = case shown="True" w621 {
              tunnel: "Cap 1 T ON" -> [w623 w624]
              frame False {
                n327 = property on="Trap 1 (ON/OFF)" class="Bool (strict)"("Val(Sgnl)"=w623) -> ()  [unwired: 2 in, 2 out]
              }
              frame True {
                n328 = property on="Trap 2 (ON/OFF)" class="Bool (strict)"("Val(Sgnl)"=w624) -> ()  [unwired: 2 in, 2 out]
              }
            }
            n329 = property on="Got Bead 2" class="Bool"("Key Focus"=TRUE) -> ()  [unwired: 2 in, 2 out]
          }
        }
      }
      event "Move Cap. 2 (ADig Top)": Value Change {
        n330 = event-data() -> ()  [unwired: 1 in, 5 out]
        n331 = local write "Move Cap. 2 (ADig Top)"(FALSE ("Move Cap. 2 (ADig Left)")) -> ()
        n332 = flat-sequence {
          tunnel: w628 -> [w631]
          tunnel: w629 -> [w632]
          tunnel: [w632] -> w626
          tunnel: [w631] -> w625
          tunnel: w626 -> [w635]
          tunnel: w625 -> [w634]
          frame #0 {
            n333 = property on="Sample Channel\nFlow" class="Bool (strict)"("Val(Sgnl)"="Cap 2 Samp Flow ON") -> ()  [unwired: 2 in, 2 out]
          }
          frame #1 {
            w633 = FALSE ("Value (Signaling)")
            n334 = local read "Saved Stage Positions"() -> (w645:dbl[][])
            n335 = local write "Stage Moving"(TRUE ("Stage Moving")) -> ()
            n336 = Array Subset(array=w645, index (row)=1 ("index"), length (row)=1 ("length"), index (col)=1 ("index"), length (col)=3 ("length")) -> (w642:dbl[][])
            n337 = Reshape Array(w642, 3 ("dimension size")) -> (w640:dbl[])
            n338 = property on="Trap 1 (ON/OFF)" class="Bool (strict)"("Val(Sgnl)"=w633) -> ()  [unwired: 2 in, 2 out]
            n339 = property on="Trap 1 (ON/OFF)" class="Bool (strict)"("Val(Sgnl)"=w633) -> ()  [unwired: 2 in, 2 out]
            n340 = Array To Cluster(array=w640) -> (cluster=w639:cluster{"[0]":dbl, "[1]":dbl, "[2]":dbl})
            n341 = call "Set Stage Position.vi"("Position"=w639, "error in"=w634, "VISA resource name in"=w635) -> ("error out"=w638:errorcluster)  [unwired: 2 out]
            n342 = local write "Stage Control Serial Error"(w638) -> ()
          }
          frame #2 {
            n343 = local write "Stage Moving"(FALSE ("Stage Moving")) -> ()
            n344 = call <vilib>:"Beep.vi"() -> ()  [unwired: 3 in, 9 out]
            n345 = case shown="True" "Cap 2 Flow ON" {
              frame False {
              }
              frame True {
                n346 = property on="Inject Pump 3" class="Bool (strict)"("Val(Sgnl)"=TRUE ("Value (Signaling)")) -> ()  [unwired: 2 in, 2 out]
              }
            }
          }
          frame #3 {
            n347 = property on="Sample Channel\nFlow" class="Bool (strict)"("Val(Sgnl)"=FALSE ("Value (Signaling)")) -> ()  [unwired: 2 in, 2 out]
            n348 = case shown="False" "Cap. 2 BD T1?\n(ADig T1, DNA T2)" {
              tunnel: "Cap 2 T ON" -> [w654 w655]
              frame False {
                n349 = property on="Trap 2 (ON/OFF)" class="Bool (strict)"("Val(Sgnl)"=w654) -> ()  [unwired: 2 in, 2 out]
              }
              frame True {
                n350 = property on="Trap 1 (ON/OFF)" class="Bool (strict)"("Val(Sgnl)"=w655) -> ()  [unwired: 2 in, 2 out]
              }
            }
            n351 = property on="Got Bead 1" class="Bool"("Key Focus"=TRUE) -> ()  [unwired: 2 in, 2 out]
          }
        }
      }
      event "Send string\nto Blue Laser": Value Change {
        n352 = event-data() -> ()  [unwired: 1 in, 5 out]
        n353 = flat-sequence {
          tunnel: w656 -> [w657]
          frame #0 {
            n354 = call "serial write macro.vi"("String"="command string", "Delay (ms)"="Delay (ms)", "VISA resource name"=w657) -> ("read buffer"=→"read blue buffer":string, "error out"=→"Blue Error Out":errorcluster)  [unwired: 1 out]
            "command string sent" <- "command string"
          }
          frame #1 {
            n355 = local write "Send string\nto Blue Laser"(FALSE ("Send string")) -> ()
          }
        }
      }
      event "Get Blue Laser State": Value Change {
        n356 = event-data() -> ()  [unwired: 1 in, 5 out]
        n357 = local read "Delay (ms)"() -> (w664:i32)
        n358 = flat-sequence {
          tunnel: w664 -> [w672]
          tunnel: w663 -> [w675]
          tunnel: [w673] -> w668
          tunnel: [w672] -> w667
          tunnel: [w682] -> w666
          tunnel: [w679] -> w665
          tunnel: w668 -> [w680]
          tunnel: w667 -> [w679]
          tunnel: w666 -> [w688]
          tunnel: w665 -> [w686]
          frame #0 {
            w670 = "l?"
            n359 = local write "command string sent"(w670) -> ()
            n360 = call "serial write macro.vi"("String"=w670, "Delay (ms)"=w672, "VISA resource name"=w675) -> ("read buffer"=w671:string, "VISA resource name out"=w673:refnum<visa-resource-name>)  [unwired: 1 out]
            n361 = Decimal String To Number(string=w671) -> (number=w674:i32)  [unwired: 2 in, 1 out]
            n362 = Not Equal To 0?(x=w674) -> (x != 0?=→"Laser On":bool)
            n363 = local write "read blue buffer"(w671) -> ()
          }
          frame #1 {
            w677 = "games?" ("String")
            n364 = local write "command string sent"(w677) -> ()
            n365 = call "serial write macro.vi"("String"=w677, "Delay (ms)"=w679, "VISA resource name"=w680) -> ("read buffer"=w678:string, "VISA resource name out"=w682:refnum<visa-resource-name>)  [unwired: 1 out]
            n366 = Decimal String To Number(string=w678) -> (number=w681:i32)  [unwired: 2 in, 1 out]
            n367 = local write "read blue buffer"(w678) -> ()
            n368 = Not Equal To 0?(x=w681) -> (x != 0?=→"Analog Modulation":bool)
          }
          frame #2 {
            w684 = "gdmes?" ("String")
            n369 = local write "command string sent"(w684) -> ()
            n370 = call "serial write macro.vi"("String"=w684, "Delay (ms)"=w686, "VISA resource name"=w688) -> ("read buffer"=w685:string)  [unwired: 2 out]
            n371 = Decimal String To Number(string=w685) -> (number=w687:i32)  [unwired: 2 in, 1 out]
            n372 = Not Equal To 0?(x=w687) -> (x != 0?=→"Digital Modulation":bool)
            n373 = local write "read blue buffer"(w685) -> ()
          }
          frame #3 {
            n374 = local write "Get Blue Laser State"(FALSE) -> ()
          }
        }
      }
      event "Blue Laser Power (mW)\n(Constant Power Mode)", "Blue Laser Modulation\nPower (mW)": Value Change {
        n375 = event-data() -> ()  [unwired: 1 in, 5 out]
        n376 = flat-sequence {
          tunnel: w691 -> [w697]
          tunnel: [w695] -> w690
          tunnel: w690 -> [w704]
          frame #0 {
            n377 = local read "Delay (ms)"() -> (w696:i32)
            n378 = Concatenate Strings("slmp " ("string"), "Blue Laser Modulation\nPower (mW)") -> (w692:string)
            n379 = call "serial write macro.vi"("String"=w692, "Delay (ms)"=w696, "VISA resource name"=w697) -> ("read buffer"=w693:string, "error out"=w694:errorcluster, "VISA resource name out"=w695:refnum<visa-resource-name>)
            n380 = local write "command string sent"(w692) -> ()
            n381 = local write "read blue buffer"(w693) -> ()
            n382 = local write "Blue Error Out"(w694) -> ()
          }
          frame #1 {
            n383 = local read "Delay (ms)"() -> (w703:i32)
            n384 = Concatenate Strings("p " ("string"), "Blue Laser Power (mW)\n(Constant Power Mode)") -> (w700:string)
            n385 = call "serial write macro.vi"("String"=w700, "Delay (ms)"=w703, "VISA resource name"=w704) -> ("read buffer"=w701:string, "error out"=w702:errorcluster)  [unwired: 1 out]
            n386 = local write "command string sent"(w700) -> ()
            n387 = local write "read blue buffer"(w701) -> ()
            n388 = local write "Blue Error Out"(w702) -> ()
          }
        }
      }
      event "Laser interlacing mode", "Blue Laser Modulation Mode", "Blue Laser ON": Value Change {
        n389 = event-data() -> ()  [unwired: 1 in, 5 out]
        n390 = flat-sequence {
          tunnel: w710 -> [w715]
          tunnel: [w714] -> w707
          tunnel: [w720] -> w709
          tunnel: w707 -> [w723]
          tunnel: w709 -> [w735]
          tunnel: [w729] -> w708
          tunnel: w708 -> [w742]
          frame #0 {
            n391 = local read "Blue Laser ON"() -> (w712:bool)
            n392 = local read "Delay (ms)"() -> (w713:i32)
            n393 = case shown="False" w712 {
              tunnel: ["l0" "l1"] -> w711
              frame False {
              }
              frame True {
              }
            }
            n394 = call "serial write macro.vi"("String"=w711, "Delay (ms)"=w713, "VISA resource name"=w715) -> ("error out"=w716:errorcluster, "VISA resource name out"=w714:refnum<visa-resource-name>)  [unwired: 1 out]
            n395 = local write "Blue Error Out"(w716) -> ()
          }
          frame #1 {
            n396 = local read "Laser interlacing mode"() -> (w725:enum32{"Laser ON", "Laser OFF", "Interlace"})
            n397 = case shown="\"Laser ON\"" w725 {
              tunnel: ["cp" "em" "l0"] -> w719
              frame "Laser ON" {
              }
              frame "Interlace" {
              }
              frame "Laser OFF", Default {
              }
            }
            n398 = local read "Delay (ms)"() -> (w724:i32)
            n399 = call "serial write macro.vi"("String"=w719, "Delay (ms)"=w724, "VISA resource name"=w723) -> ("read buffer"=w721:string, "error out"=w722:errorcluster, "VISA resource name out"=w720:refnum<visa-resource-name>)
            n400 = local write "command string sent"(w719) -> ()
            n401 = local write "read blue buffer"(w721) -> ()
            n402 = local write "Blue Error Out"(w722) -> ()
          }
          frame #2 {
            n403 = case shown="\"Analog Modulation\"" "Blue Laser Modulation Mode" {
              tunnel: ["sdmes 0" "sdmes 1" "sdmes 1"] -> w730
              frame "Analog Modulation" {
              }
              frame "Digital + Analog Modulation" {
              }
              frame "Digital Modulation", Default {
              }
            }
            n404 = local read "Delay (ms)"() -> (w733:i32)
            n405 = call "serial write macro.vi"("String"=w730, "Delay (ms)"=w733, "VISA resource name"=w735) -> ("read buffer"=w731:string, "error out"=w732:errorcluster, "VISA resource name out"=w729:refnum<visa-resource-name>)
            n406 = local write "command string sent"(w730) -> ()
            n407 = local write "read blue buffer"(w731) -> ()
            n408 = local write "Blue Error Out"(w732) -> ()
          }
          frame #3 {
            n409 = local read "Blue Laser Modulation Mode"() -> (w744:string)
            n410 = case shown="\"Digital Modulation\", Default" w744 {
              tunnel: ["sames 1" "sames 1" "sames 0"] -> w740
              frame "Analog Modulation" {
              }
              frame "Digital + Analog Modulation" {
              }
              frame "Digital Modulation", Default {
              }
            }
            n411 = local read "Delay (ms)"() -> (w743:i32)
            n412 = local write "command string sent"(w740) -> ()
            n413 = call "serial write macro.vi"("String"=w740, "Delay (ms)"=w743, "VISA resource name"=w742) -> ("read buffer"=w741:string, "error out"=w739:errorcluster)  [unwired: 1 out]
            n414 = local write "read blue buffer"(w741) -> ()
            n415 = local write "Blue Error Out"(w739) -> ()
          }
        }
      }
      event "Read Harvard": Value Change {
        n416 = event-data() -> ()  [unwired: 1 in, 5 out]
        n417 = Concatenate Strings("write buffer", "\r") -> (w752:string)
        n418 = VISA Write(VISA resource name=w750, write buffer=w752, error in (no error)=w749) -> (VISA resource name out=w761:refnum<visa-resource-name>, error out=w760:errorcluster)  [unwired: 1 out]
        n419 = stacked-sequence {
          tunnel: [w764] -> w759
          tunnel: w761 -> [w764]
          tunnel: w760 -> [w763]
          tunnel: [w763] -> w754
          frame #0 {
            n420 = Wait (ms)(milliseconds to wait=50) -> ()  [unwired: 1 out]
          }
        }
        n421 = property class="Instr"(reference=w759, error in=w754) -> (reference out=w758:refnum<visa-resource-name>, error out=w756:errorcluster, "Serial Settings:Number of Bytes at Serial Port"=w757:u32)
        "Serial Settings:Number of Bytes at Serial Port" <- w757
        n422 = VISA Read(VISA resource name=w758, byte count=w757, error in (no error)=w756) -> (read buffer=w755:string)  [unwired: 3 out]
        "read buffer" <- w755
        n423 = Fract/Exp String To Number(string=w755) -> ()  [unwired: 5 out]
      }
      event "+z", "-z": Value Change {
        n424 = event-data() -> ()  [unwired: 1 in, 5 out]
        n425 = flat-sequence {
          tunnel: w765 -> [w787]
          tunnel: w766 -> [w767]
          frame #0 {
            n426 = call "Read Stage Position.vi"("error in"=w787, "VISA resource name in"=w767) -> ("Current Position"=w772:cluster{dbl, dbl, dbl}, "error out"=w785:errorcluster, "VISA resource name out"=w786:refnum<visa-resource-name>)  [unwired: 1 out]
            n427 = local read "Saved Stage Positions"() -> (w796:dbl[][])
            n428 = Divide(x="z nudge increment (um)", y=1000.0) -> (x/y=w784:dbl)
            n429 = Boolean To (0,1)(Boolean="+z") -> (0, 1=w776:i16)
            n430 = Boolean To (0,1)(Boolean="-z") -> (0, 1=w777:i16)
            n431 = Array Subset(array=w796, index (row)=1 ("index"), length (row)=1 ("length"), index (col)=1 ("index"), length (col)=3 ("length")) -> (w793:dbl[][])
            n432 = Multiply(x=w776, y=w784) -> (x*y=w780:dbl)
            n433 = Multiply(x=w777, y=w784) -> (x*y=w778:dbl)
            n434 = Unbundle(w772) -> (w770:dbl, w769:dbl, w773:dbl)
            n435 = Negate(x=w778) -> (-x=w779:dbl)
            n436 = Reshape Array(w793, 3 ("dimension size")) -> (w791:dbl[])
            n437 = Add(x=w780, y=w779) -> (x+y=w781:dbl)
            n438 = Array To Cluster(array=w791) -> ()  [unwired: 1 out]
            n439 = Add(x=w781, y=w773) -> (x+y=w771:dbl)
            n440 = Bundle(cluster=w772, w770, w769, w771) -> (w768:cluster{dbl, dbl, dbl})
            n441 = call "Set Stage Position.vi"("Position"=w768, "error in"=w785, "VISA resource name in"=w786) -> ("error out"=w790:errorcluster)  [unwired: 2 out]
            n442 = local write "Stage Moving"(TRUE ("Stage Moving")) -> ()
            n443 = local write "Stage Control Serial Error"(w790) -> ()
          }
          frame #1 {
            n444 = local write "Stage Moving"(FALSE ("Stage Moving")) -> ()
          }
        }
      }
      event "-y", "+y": Value Change {
        n445 = event-data() -> ()  [unwired: 1 in, 5 out]
        n446 = flat-sequence {
          tunnel: w799 -> [w823]
          tunnel: w800 -> [w806]
          frame #0 {
            n447 = call "Read Stage Position.vi"("error in"=w823, "VISA resource name in"=w806) -> ("Current Position"=w809:cluster{dbl, dbl, dbl}, "error out"=w821:errorcluster, "VISA resource name out"=w822:refnum<visa-resource-name>)  [unwired: 1 out]
            n448 = Divide(x="y nudge increment (um", y=1000.0) -> (x/y=w820:dbl)
            n449 = Boolean To (0,1)(Boolean="+y") -> (0, 1=w812:i16)
            n450 = Boolean To (0,1)(Boolean="-y") -> (0, 1=w813:i16)
            n451 = Multiply(x=w812, y=w820) -> (x*y=w816:dbl)
            n452 = Multiply(x=w813, y=w820) -> (x*y=w814:dbl)
            n453 = Unbundle(w809) -> (w808:dbl, w803:dbl, w805:dbl)
            n454 = Negate(x=w814) -> (-x=w815:dbl)
            n455 = Add(x=w816, y=w815) -> (x+y=w817:dbl)
            n456 = Add(x=w817, y=w803) -> (x+y=w804:dbl)
            n457 = Bundle(cluster=w809, w808, w804, w805) -> (w807:cluster{dbl, dbl, dbl})
            n458 = call "Set Stage Position.vi"("Position"=w807, "error in"=w821, "VISA resource name in"=w822) -> ("error out"=w802:errorcluster)  [unwired: 2 out]
